vi "CastToMoreSpecificClass.vi"(11 "Sequence Context In":refnum<k7>) -> (0 "error out":errorcluster, 2 "Seconds Executing":dbl, 3 "Result Status":string)   [LabVIEW 2011]
doc: "This VI demonstrates how to cast to a more specific class to access the properties or methods of that class."
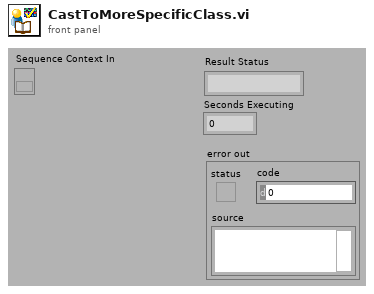
[diagram p1: front panel]
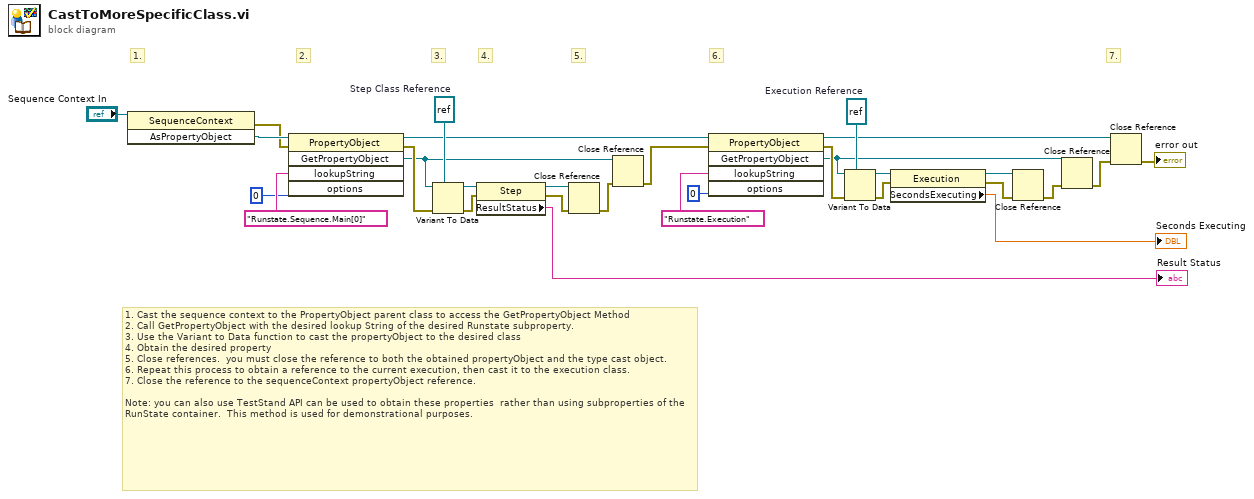
[diagram p0: block diagram]
diagram:
  w21 = refnum<k7> refnum  # Execution Reference
  w27 = refnum<k7> refnum  # Step Class Reference
  # "7."
  # "6."
  # "5."
  # "4."
  # "3."
  # "2."
  # "1."
  # "1. Cast the sequence context to the PropertyObject parent class to access the GetPropertyObject Method\n2. Call GetPropertyObject with the desired lookup String of the desired Runstate subproperty.  \n3. Use the Variant to Data function to cast the propertyObject to the desired class\n4. Obtain the desired property\n5. Close references.  you must close the reference to both the obtained propertyObject and the type cast object.\n6. Repeat this process to obtain a reference to the current execution, then cast it to the execution class.\n7. Close the reference to the sequenceContext propertyObject reference. \n\nNote: you can also use TestStand API can be used to obtain these properties  rather than using subproperties of the RunState container.  This method is used for demonstrational purposes."
  n1 = invoke class="SequenceContext" method="AsPropertyObject"(reference="Sequence Context In") -> (error out=w22:errorcluster, "AsPropertyObject"=w23:refnum<k7>)  [unwired: 2 in, 1 out]
  n2 = invoke class="PropertyObject" method="GetPropertyObject"(reference=w23, error in=w22, "lookupString"="Runstate.Sequence.Main[0]", "options"=0) -> (reference out=w3:refnum<k7>, error out=w17:errorcluster, "GetPropertyObject"=w6:refnum<k7>)  [unwired: 1 in, 2 out]
  n3 = Variant To Data(error in=w17, type=w27, Variant=w6) -> (data=w26:refnum<k7>, error out=w18:errorcluster)
  n4 = property class="Step"(reference=w26, error in=w18) -> (reference out=w12:refnum<k7>, error out=w13:errorcluster, "ResultStatus"=→"Result Status":string)
  n5 = Close Reference(reference=w12, error in (no error)=w13) -> (error out=w9:errorcluster)
  n6 = Close Reference(reference=w6, error in (no error)=w9) -> (error out=w4:errorcluster)
  n7 = invoke class="PropertyObject" method="GetPropertyObject"(reference=w3, error in=w4, "lookupString"="Runstate.Execution", "options"=0) -> (reference out=w1:refnum<k7>, error out=w20:errorcluster, "GetPropertyObject"=w7:refnum<k7>)  [unwired: 1 in, 2 out]
  n8 = Variant To Data(error in=w20, type=w21, Variant=w7) -> (data=w16:refnum<k7>, error out=w19:errorcluster)
  n9 = property class="Execution"(reference=w16, error in=w19) -> (reference out=w10:refnum<k7>, error out=w11:errorcluster, "SecondsExecuting"=→"Seconds Executing":dbl)
  n10 = Close Reference(reference=w10, error in (no error)=w11) -> (error out=w8:errorcluster)
  n11 = Close Reference(reference=w7, error in (no error)=w8) -> (error out=w2:errorcluster)
  n12 = Close Reference(reference=w1, error in (no error)=w2) -> (error out=→"error out":errorcluster)
